vi "MGI Get Detail and Call Chain[].vi"(7 "MGI Error Reporter Base In":refnum<class "MGI Error Reporter Base.lvclass">, 11 "MGI ERD LB Row Base in":refnum<class "MGI ERD LB Row Base.lvclass">) -> (1 "Call Chain[..Top Level]":string[](array[string]), 2 "Details":string)   [LabVIEW 2020, in "MGI ERD LB Row Base.lvclass"]
doc: "Authored by Shawn Walpole\nsupport@mooregoodideas.com\nwww.mooregoodideas.com\n\nCopyright (c) 2013, Moore Good Ideas, Inc.\n\nAll rights reserved.\n\nRedistribution and use in source and binary forms, with or without modification, are permitted provided that the following conditions are met:\n\n * Redistributions of source code must retain the above copyright notice, this list of conditions and the following disclaimer.\n * Redistributions in binary form must reproduce the above copyright notice, this list of conditions and the following disclaimer in the documentation and/or other materials provided with the distribution.\n * Neither the name of Moore Good Ideas, Inc. nor the names of its contributors may be used to endorse or promote products derived from this software without specific prior written permission.\n\nTHIS SOFTWARE IS PROVIDED BY THE COPYRIGHT HOLDERS AND CONTRIBUTORS \"AS IS\" AND ANY EXPRESS OR IMPLIED WARRANTIES, INCLUDING, BUT NOT LIMITED TO, THE IMPLIED WARRANTIES OF MERCHANTABILITY AND FITNESS FOR A PARTICULAR PURPOSE ARE DISCLAIMED. IN NO EVENT SHALL THE COPYRIGHT OWNER OR CONTRIBUTORS BE LIABLE FOR ANY DIRECT, INDIRECT, INCIDENTAL, SPECIAL, EXEMPLARY, OR CONSEQUENTIAL DAMAGES (INCLUDING, BUT NOT LIMITED TO, PROCUREMENT OF SUBSTITUTE GOODS OR SERVICES; LOSS OF USE, DATA, OR PROFITS; OR BUSINESS INTERRUPTION) HOWEVER CAUSED AND ON ANY THEORY OF LIABILITY, WHETHER IN CONTRACT, STRICT LIABILITY, OR TORT (INCLUDING NEGLIGENCE OR OTHERWISE) ARISING IN ANY WAY OUT OF THE USE OF THIS SOFTWARE, EVEN IF ADVISED OF THE POSSIBILITY OF SUCH DAMAGE."
uses:
  <userlib>/_MGI/Error Reporter/MGI Error Reporter Dialog/MGI ERD LB Row Base/MGI ERD LB Row Base.lvclass
  <userlib>/_MGI/Error Reporter/MGI Error Reporter Base/MGI Error Reporter Base.lvclass
  <vilib>/Utility/error.llb/DialogType.ctl
  <userlib>/_MGI/Error Reporter/MGI Error Reporter Dialog/MGI ERD LB Row Base/MGI ERD LB Row Base.lvclass/MGI ERD LB Row Base.ctl
  <vilib>/Utility/error.llb/whitespace.ctl
panel:
  # "-1073807194"
  # "-1073807298"
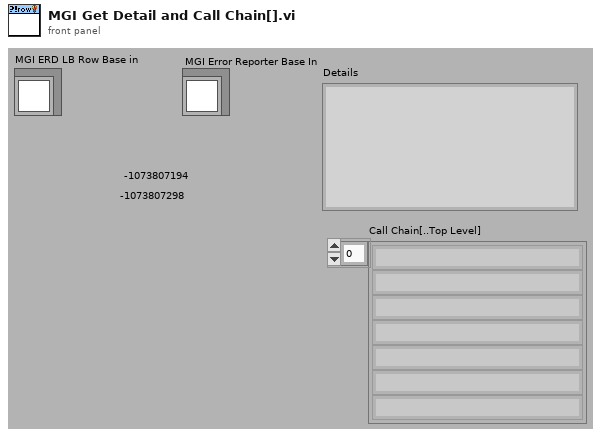
[diagram p1: front panel]
types:
  T1 = typedef "DialogType.ctl" = u16
  T2 = typedef "whitespace.ctl" = u16
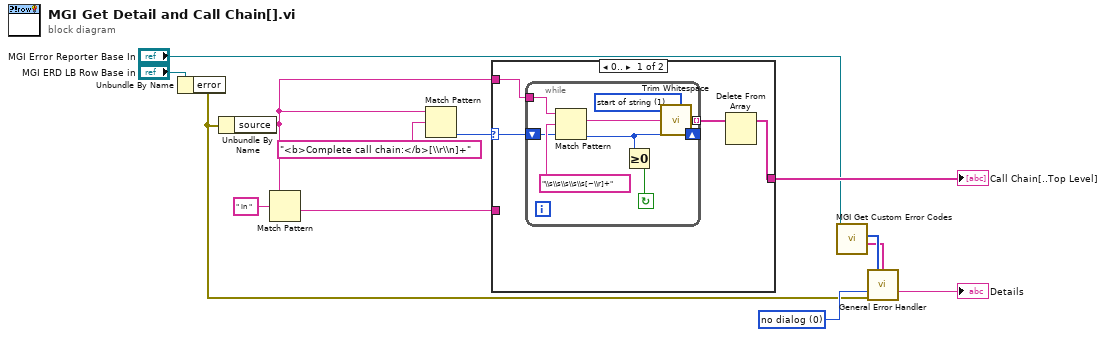
[diagram p0: block diagram]
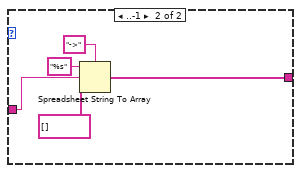
[diagram p2: hidden frame]
diagram:
  w13 = T1 0 items=["no dialog", "OK message", "continue or stop message", "OK message + warnings", "continue/stop + warnings"] ("type of dialog (OK msg:1)")
  n1 = Unbundle By Name("MGI ERD LB Row Base in") -> ("error"=w4:errorcluster)
  n2 = Unbundle By Name(w4) -> ("source"=w2:string)
  n3 = Match Pattern(string=w2, regular expression=" in " ("search string/char (-)")) -> (after substring=w3:string)  [unwired: 4 out]
  n4 = Match Pattern(string=w2, regular expression="<b>Complete call chain:</b>[\\r\\n]+") -> (offset past match=w8:i32)  [unwired: 4 out]
  n5 = case shown="0.." w8 {
    selector: w8 -> [w16 _]
    tunnel: w2 -> [w17 _]
    tunnel: w3 -> [_ w30]
    tunnel: [w14 w29] -> w7
    frame 0.. {
      n6 = while {
        tunnel: w17 -> [w22]
        shift-right: [w21] -> _
        shift-left: w16 -> [w23]
        tunnel: [w18] -> w15 mode=indexing
        stop <- w24 continue-if-true
        w19 = T2 1 items=["both", "start of string", "end of string"] ("location (both)")
        n7 = Match Pattern(string=w22, regular expression="\\s\\s\\s\\s\\s[~\\r]+", offset (0)=w23) -> (match substring=w20:string, offset past match=w21:i32)  [unwired: 2 out]
        n8 = Greater Or Equal To 0?(x=w21) -> (x >= 0?=w24:bool)
        n9 = call <vilib>:"Trim Whitespace.vi"("string"=w20, "location (both)"=w19) -> ("trimmed string"=w18:string)
      }
      n10 = Delete From Array(array=w15) -> (array with subset deleted=w14:string[])  [unwired: 2 in, 1 out]
    }
    frame ..-1 {
      n11 = Spreadsheet String To Array(delimiter (Tab)="->", format string="%s", spreadsheet string=w30, array type (2D Dbl)=string[] []) -> (array=w29:string[])
    }
  }
  "Call Chain[..Top Level]" <- w7
  n12 = call-dynamic "MGI Get Custom Error Codes.vi"("MGI Error Reporter Base In"="MGI Error Reporter Base In") -> ("Custom Name[]"=w11:string[], "Custom Code[]"=w12:i32[])  [unwired: 9 out]
  n13 = call <vilib>:"General Error Handler.vi"("[user-defined codes]"=w12, "[user-defined descriptions]"=w11, "type of dialog (OK msg:1)"=w13, "error in (no error)"=w4) -> ("message"=→"Details":string)  [unwired: 1 in, 10 out]
